vi "LinxGetDeviceId.vi"(8 "Error In":errorcluster, 11 "LINX Resource":T1) -> (0 "Error Out":errorcluster, 2 "DeviceID":u8, 3 "LINX Resource":T1)   [LabVIEW 2014, in "LMH-LINX.lvlib" / "Local IO.lvlib"]
uses:
  <vilib>/MakerHub/LINX/Private/Local IO/Local IO.lvlib
  <vilib>/MakerHub/LINX/Private/Type Defs/LINX Ref.ctl
  <vilib>/MakerHub/LINX/Private/Type Defs/Platform.ctl
  <vilib>/MakerHub/LINX/Private/Type Defs/Interface.ctl
  <vilib>/MakerHub/LINX/Private/Device/Type Defs/LINX Device Config.ctl
  <vilib>/MakerHub/LINX/Private/Device/Type Defs/TCP Config.ctl
  <vilib>/MakerHub/LINX/Private/Device/Type Defs/Channels.ctl
  <vilib>/MakerHub/LINX/Private/Type Defs/Error Type.ctl
  <vilib>/MakerHub/LINX/LMH-LINX.lvlib
  liblinxdevice.dll
  <vilib>/MakerHub/LINX/Private/Device/Device.lvlib
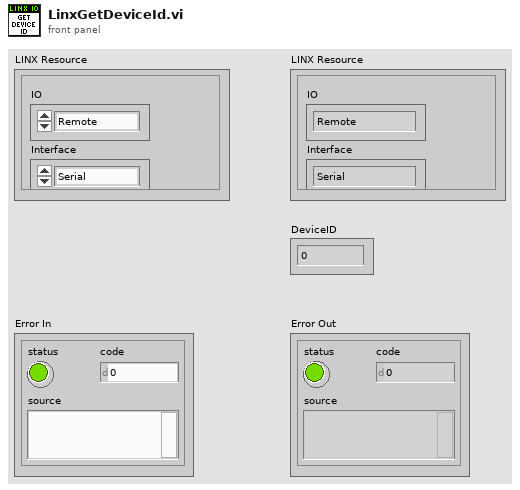
[diagram p1: front panel]
types:
  T1 = typedef "LMH-LINX.lvlib/LINX Ref.ctl" = cluster{"IO":T2, "Interface":T3, "LINX Device Config":T4}
  T2 = typedef "LMH-LINX.lvlib/Platform.ctl" = enum16{"Remote", "Local"}
  T3 = typedef "LMH-LINX.lvlib/Interface.ctl" = enum16{"Serial", "TCP"}
  T4 = typedef "LMH-LINX.lvlib/Device.lvlib/LINX Device Config.ctl" = cluster{"Interface":T3, "COM Port":refnum<visa-resource-name>, "TCP Configuration":T5, "Device Family":u8, "Device ID":u8, "Device Name":string, "TCP Ref":refnum<k5>, "Channels":T6}
  T5 = typedef "LMH-LINX.lvlib/Device.lvlib/TCP Config.ctl" = cluster{"IP Address":string, "Port":u16}
  T6 = typedef "LMH-LINX.lvlib/Channels.ctl" = cluster{"DI":u8[], "DO":u8[], "AI":u8[], "AO":u8[], "PWM":u8[], "QE":u8[], "UART":u8[], "I2C 2":u8[], "SPI":u8[], "CAN":u8[], "Servo":u8[], "AI Ref (V)":dbl, "AI Resolution (Bits)":u8, "AO Ref (V)":dbl, "AO Resolution (Bits)":u8}
  T7 = typedef "LMH-LINX.lvlib/Error Type.ctl" = enum16{"Unknown", "Timeout", "Corrupt Return Packet", "Unable To Connect", "Command Not Supported", "Channel DNE", "Invalid COM Config", "Firmware Version Mismatch", "myRIO Support", "CMD Specific Error", "Local IO Not Supported"}
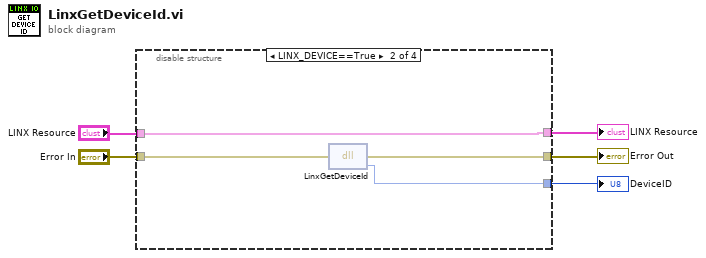
[diagram p0: block diagram]
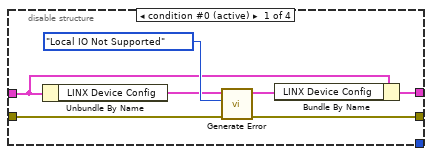
[diagram p2: hidden frame]
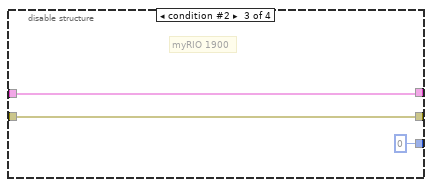
[diagram p3: hidden frame]
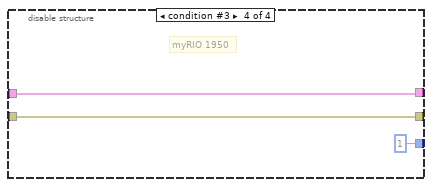
[diagram p4: hidden frame]
diagram:
  n1 = disable-structure shown="LINX_DEVICE==True" {
    disable-tunnel: [w6 w16 w18 w21] -> w2
    disable-tunnel: "LINX Resource" -> [w8 w16 w18 w21]
    disable-tunnel: "Error In" -> [w11 w15 w19 w22]
    disable-tunnel: [w10 w14 w19 w22] -> w3
    disable-tunnel: [_ w13 u8 0 ("DeviceFamily") u8 1 ("DeviceFamily")] -> w1
    frame condition #0 (active) {
      n2 = Unbundle By Name(w8) -> ("LINX Device Config"=w9:T4)
      n3 = call <vilib>:"Generate Error.vi"("Error In"=w11, "Error Type"=Error_Type."Local IO Not Supported", "LINX Device Config"=w9) -> ("Error Out"=w10:errorcluster, "Dup LINX Device Config"=w7:T4)  [unwired: 7 in]
      n4 = Bundle By Name(cluster=w8, "LINX Device Config"=w7) -> (w6:T1)
    }
    frame condition #1 {
      n5 = dll-call lib="liblinxdevice.*" fn="LinxGetDeviceId"(error in=w15) -> (error out=w14:errorcluster, "DeviceId"=w13:u8)  [unwired: 2 in, 1 out]
    }
    frame condition #2 {
      # "myRIO 1900"
    }
    frame condition #3 {
      # "myRIO 1950"
    }
  }
  "Error Out" <- w3
  "LINX Resource" <- w2
  "DeviceID" <- w1
